vi "Create image array.vi"(8 "error in (no error)":errorcluster, 11 "Name idx":string[](array[string])) -> (0 "error out":errorcluster, 3 "Image array":T1[](array[typedef]))   [LabVIEW 2020]
doc: "Create an image array where Name idx is a list of names for each image. Every image name is added with a unique ID to avoid replicates."
uses:
  <vilib>/vision/Image Controls.llb/IMAQ Image.ctl
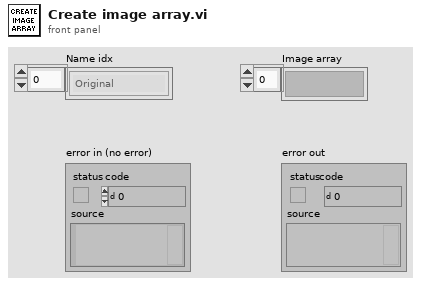
[diagram p1: front panel]
types:
  T1 = typedef "IMAQ Image.ctl" = refnum<image>
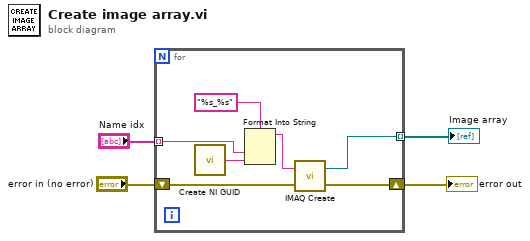
[diagram p0: block diagram]
diagram:
  n1 = for {
    shift-right: [w11] -> w4
    shift-left: "error in (no error)" -> [w10]
    tunnel: "Name idx" -> [w6] mode=indexing
    tunnel: [w5] -> w1 mode=indexing
    n2 = call <vilib>:"Create NI GUID.vi"() -> ("NI GUID"=w8:string)
    n3 = Format Into String(format string="%s_%s", w6, w8) -> (resulting string=w9:string)  [unwired: 2 in, 1 out]
    n4 = call "IMAQ Create"("Image Name"=w9, "error in (no error)"=w10) -> ("New Image"=w5:T1, "error out"=w11:errorcluster)  [unwired: 3 in]
  }
  "error out" <- w4
  "Image array" <- w1
